vi "Update Status Message for Test.vi"(11 "MTS Temp Sensor Test in":refnum<class "MTS Temp Sensor Test.lvclass">) -> ()   [LabVIEW 2015, in "MTS Temp Sensor Test.lvclass"]
uses:
  MTS Temp Sensor Test.lvclass
  Test Class/Test Class.lvclass
  Classes/Application/Class/Application.lvclass
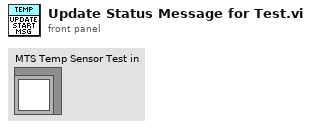
[diagram p1: front panel]
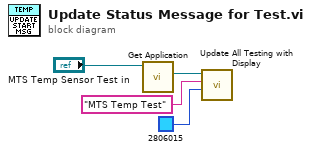
[diagram p0: block diagram]
diagram:
  n1 = call "Get Application.vi"("Test Class in"="MTS Temp Sensor Test in") -> ("Application.lvlib:Application.lvclass"=w4:refnum<class "Application.lvclass">)  [unwired: 9 in, 1 out]
  n2 = call "Update All Testing with Display.vi"("BG Color"=u32 2806015, "Message ('')"="MTS Temp Test", "Application in"=w4) -> ()  [unwired: 7 in, 2 out]
